vi "2ndHiddenLayerANN.vi"(10 "2nd HiddenIn":sgl[](array[numeric])=[0.0, 0.0, 0.0, 0.0]) -> (3 "2ndHiddenOut":sgl[](array[numeric]))   [LabVIEW 2020]
uses:
  <vilib>/rvi/Memory/Memory_Emulation/nirvimemoryFastEmulation.vi
  <vilib>/rvi/Memory/Memory_Emulation/nirvimemoryEmulation.vi
  <vilib>/rvi/Emulation/niFpgaEmulationIsFPGAContextNoSignature.vi
  <vilib>/rvi/DataTransferAndStorage/Container/Common/niFpgaContainerGetUniqueNameForEmu.vi
  <vilib>/rvi/Emulation/niFpgaProcessEmulError.vi
  <vilib>/rvi/Emulation/niFpgaSctlEmulationGetInTimedLoop.vi
  <vilib>/rvi/errors/nirviReportUnexpectedCaseInternalError (U32).vi
  <vilib>/rvi/DataTransferAndStorage/Container/XNode/niFpgaContainer.xnode
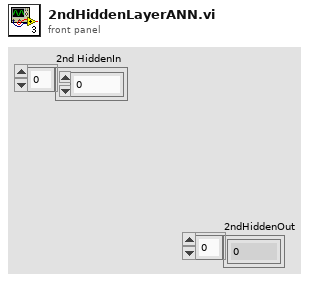
[diagram p1: front panel]
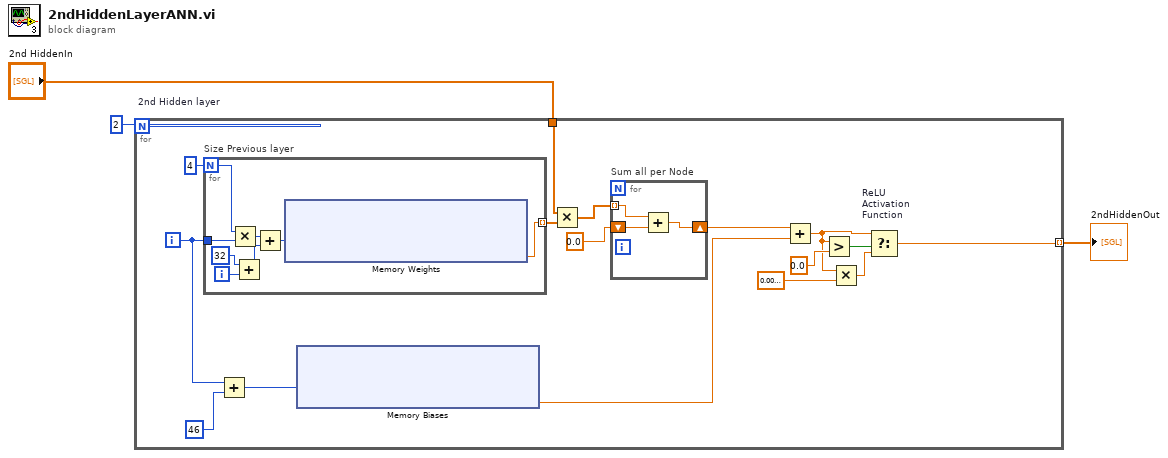
[diagram p0: block diagram]
diagram:
  w2 = 2  # 2nd Hidden layer
  n1 = for {
    N: w2 -> [_]
    tunnel: "2nd HiddenIn" -> [w15]
    tunnel: [w7] -> w1 mode=indexing
    i -> [w12]
    n2 = for "Size Previous layer" {
      N: 4 ("Size Previous layer") -> [w25]
      tunnel: w12 -> [w26]
      tunnel: [w27] -> w19 mode=indexing
      i -> [w22]
      n3 = Multiply(x=w25, y=w26) -> (x*y=w24:i32)
      n4 = Add(x=32, y=w22) -> (x+y=w21:i32)
      n5 = Add(x=w24, y=w21) -> (x+y=w23:i32)
      n6 = xnode "Memory Weights"("Address"=w23) -> ("Data"=w27:sgl)  [unwired: 1 in, 1 out]
    }
    n7 = Add(x=w12, y=46) -> (x+y=w14:i32)
    n8 = xnode "Memory Biases"("Address"=w14) -> ("Data"=w9:sgl)  [unwired: 1 in, 1 out]
    n9 = Multiply(x=w15, y=w19) -> (x*y=w18:sgl[])
    n10 = for "Sum all per Node" {
      tunnel: w18 -> [w30] mode=indexing
      shift-right: [w28] -> w8
      shift-left: sgl 0.0 -> [w29]
      n11 = Add(x=w30, y=w29) -> (x+y=w28:sgl)
    }
    n12 = Add(x=w8, y=w9) -> (x+y=w6:sgl)
    n13 = Greater?(x=w6, y=sgl 0.0) -> (0:w11:bool)
    n14 = Multiply(x=w6, y=sgl 0.01) -> (x*y=w4:sgl)
    n15 = Select "ReLU\nActivation\nFunction"(t=w6, s=w11, f=w4) -> (s? t:f=w7:sgl)
  }
  "2ndHiddenOut" <- w1
